vi "Search Results Panel.vi"(11 "BetterSearch in":refnum<class "BetterSearch.lvclass">) -> ()   [LabVIEW 2020, in "Better Search.lvlib" / "BetterSearch.lvclass"]
uses:
  BetterSearch.lvclass
  Search/Search.lvclass
  Data Types/Scope Options.ctl
  Data Types/Throbber.ctl
  BetterSearch.lvclass/BetterSearch.ctl
  80aabc45-af7a-4409-a262-2509359cf74b.vi
  Search Result/Search Result.lvclass
  Better Search.lvlib
panel:
  out "Throbber":T1
  out "Scope Options":T2
  in  "Results Table":i32[](listbox)
  out "Text":string
  out "Type":string
  in  "Go To":bool
  in  "Remove":bool
  out "Scope":string
  out "Launched From":string
  out "Current Search":refnum<class "Search.lvclass">
  # "Exclude"
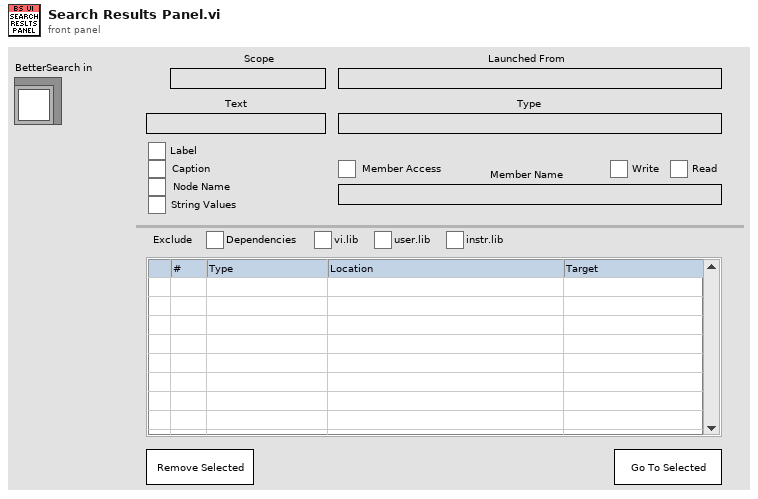
[diagram p1: front panel]
types:
  T1 = typedef "Better Search.lvlib/Throbber.ctl" = u16
  T2 = typedef "Better Search.lvlib/Scope Options.ctl" = cluster{"Include Labels":bool, "Include Captions":bool, "Include Node Name":bool, "Member Access":bool, "Member Read":bool, "Member Write":bool, "Member Name":string, "String Value":bool, "Dependencies":bool, "vi.lib":bool, "user.lib":bool, "instr.lib":bool}
  T3 = typedef "Better Search.lvlib/BetterSearch.lvclass/Results Events.ctl" = cluster{"Close Results Panel":refnum<user-event>, "Show Search":refnum<user-event>, "Show Result":refnum<user-event>, "Progress WD":refnum<user-event>}
  T4 = typedef "Better Search.lvlib/Search Params.ctl" = cluster{"Type":T5, "Type ID":string, "Text":string, "Scope":T6, "Targets":refnum<vi>[], "Scope Options":T2, "Typedef Path":path, "Member Graph Index":i32, "Member TypeID":string}
  T5 = typedef "Better Search.lvlib/Search Type.ctl" = enum16{"Generic", "Text", "Data Type", "VI", "Node"}
  T6 = typedef "Better Search.lvlib/Search Scope.ctl" = enum16{"Active Target", "Active Project", "Specific Targets", "Active VI", "Active Hierarchy"}
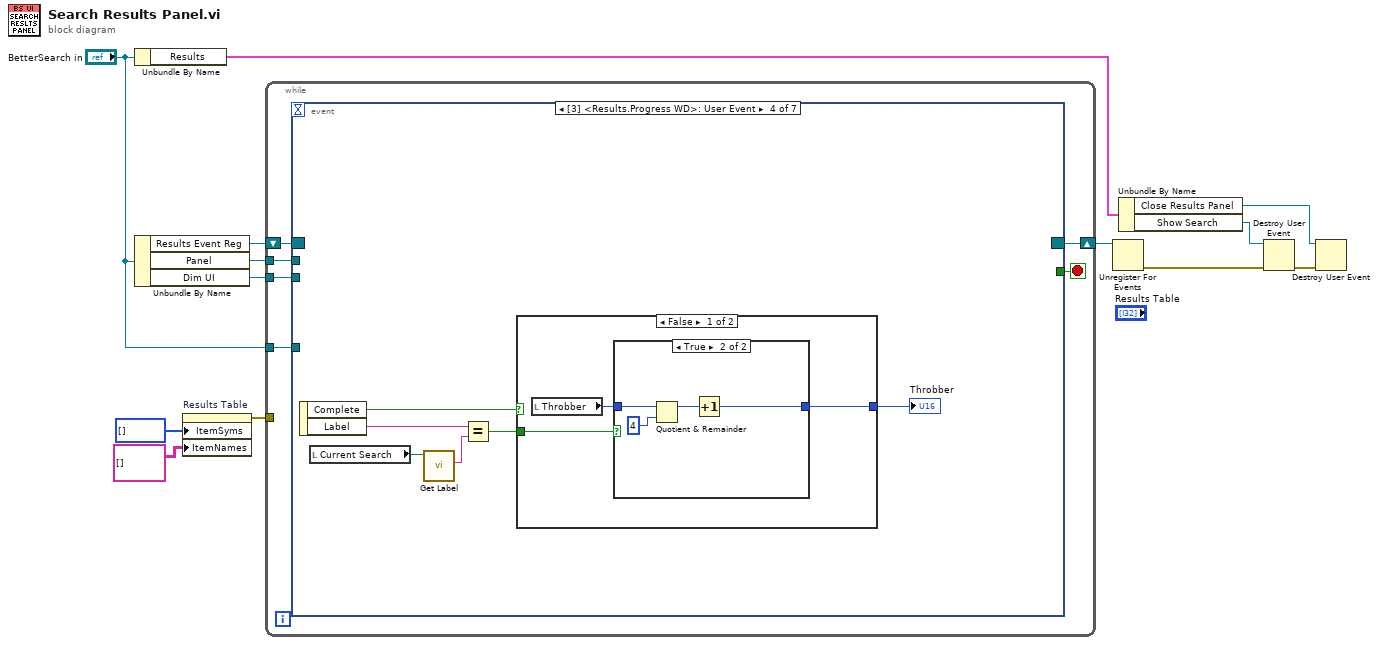
[diagram p0: block diagram]
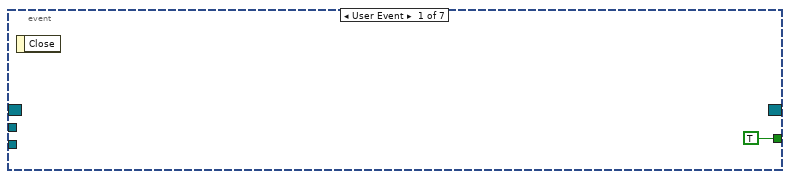
[diagram p2: hidden frame]
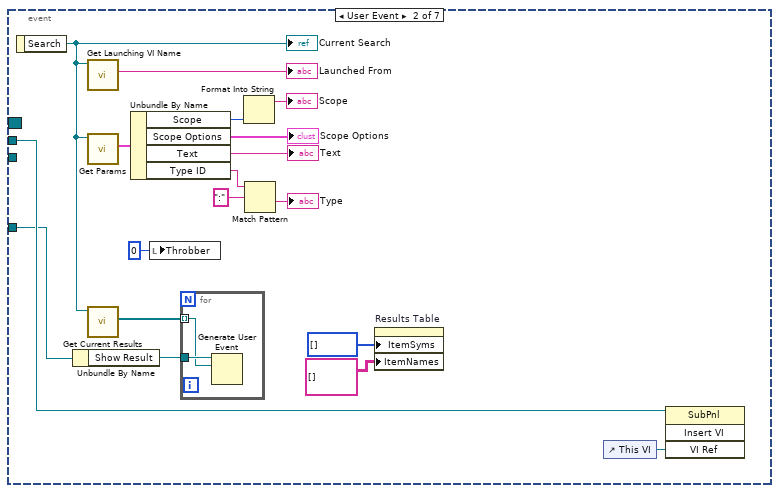
[diagram p3: hidden frame]
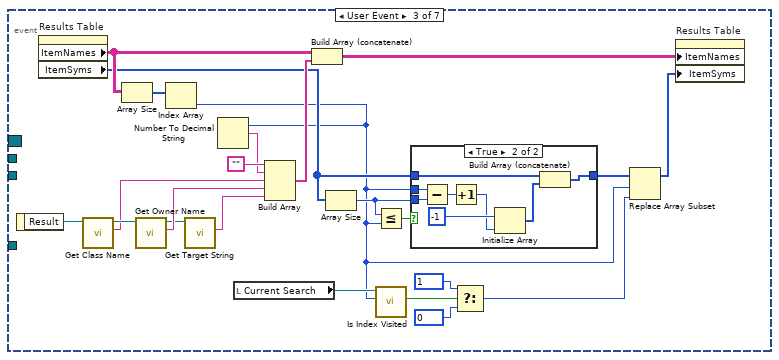
[diagram p4: hidden frame]
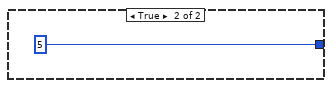
[diagram p7: hidden frame]
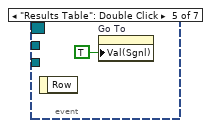
[diagram p8: hidden frame]
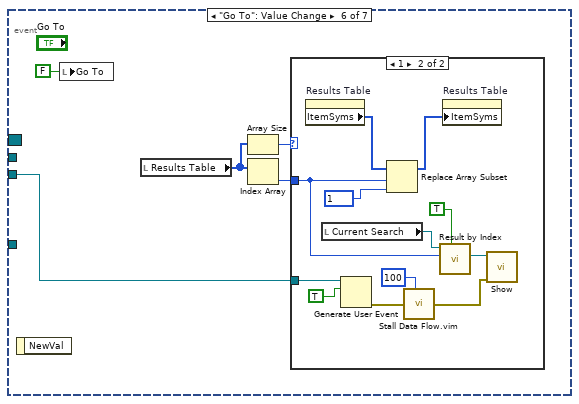
[diagram p9: hidden frame]
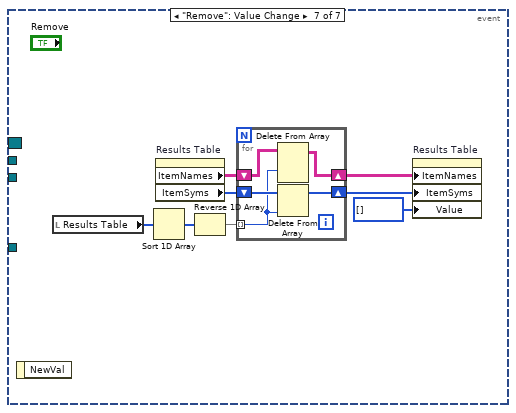
[diagram p11: hidden frame]
diagram:
  n1 = Unbundle By Name("BetterSearch in") -> ("Results"=w9:T3)
  n2 = Unbundle By Name("BetterSearch in") -> ("Results Event Reg"=w13:refnum<event-registration>, "Panel"=w6:refnum<vi>, "Dim UI"=w3:refnum<user-event>)
  n3 = property on="Results Table" class="MCListbox (strict)"("ItemSyms"=i32[] [] ("Item Symbols"), "ItemNames"=string[][] [] ("Item Names")) -> (error out=w2:errorcluster)  [unwired: 2 in, 1 out]
  n4 = while {
    shift-right: [w18] -> w12
    shift-left: w13 -> [w19]
    tunnel: w6 -> [w16]
    tunnel: w3 -> [w15]
    tunnel: w2 -> [_]
    tunnel: "BetterSearch in" -> [w14]
    stop <- w17 stop-if-true
    n5 = event shown="[3] <Results.Progress WD>: User Event" {
      selector: w19 -> [_ _ _ _ _ _ _]
      dyn-events: [_ _ _ _ _ _ _] -> w18
      timeout: _ -> [_ _ _ _ _ _ _]
      tunnel: [TRUE _ _ _ _ _ _] -> w17
      tunnel: w16 -> [_ w37 _ _ _ _ _]
      tunnel: w15 -> [_ _ _ _ _ w89 _]
      tunnel: w14 -> [_ w29 _ _ _ _ _]
      event User Event {
        n6 = event-data() -> ()  [unwired: 1 in, 1 out]
      }
      event User Event {
        n7 = event-data() -> ("Search"=w30:refnum<class "Search.lvclass">)  [unwired: 1 in]
        "Current Search" <- w30
        n8 = Unbundle By Name(w29) -> ("Show Result"=w28:refnum<user-event>)
        n9 = call "Get Launching VI Name.vi"("Search in"=w30) -> ("Launching VI Name"=→"Launched From":string)  [unwired: 8 in, 2 out]
        n10 = call "Get Params.vi"("Search in"=w30) -> ("Params"=w35:T4)  [unwired: 8 in, 2 out]
        n11 = call "Get Current Results.vi"("Search in"=w30) -> ("Current Results"=w27:refnum<class "Search Result.lvclass">[])  [unwired: 8 in, 2 out]
        n12 = Unbundle By Name(w35) -> ("Scope"=w34:T6, "Scope Options"=→"Scope Options":T2, "Text"=→"Text":string, "Type ID"=w25:string)
        n13 = local write "Throbber"(T1 0 ("Throbber")) -> ()
        n14 = for {
          tunnel: w28 -> [w40]
          tunnel: w27 -> [w39] mode=indexing
          n15 = Generate User Event(user event=w40, event data cluster=w39) -> ()  [unwired: 2 in, 2 out]
        }
        n16 = Format Into String(w34) -> (resulting string=→"Scope":string)  [unwired: 3 in, 1 out]
        n17 = Match Pattern(string=w25, regular expression=":") -> (after substring=→"Type":string)  [unwired: 1 in, 3 out]
        n18 = property on="Results Table" class="MCListbox (strict)"("ItemSyms"=i32[] [] ("Item Symbols"), "ItemNames"=string[][] [] ("Item Names")) -> ()  [unwired: 2 in, 2 out]
        n19 = control-ref of="This VI"() -> (w38:refnum<vi>)
        n20 = invoke class="SubPnl" method="Insert VI"(reference=w37, "VI Ref"=w38) -> ()  [unwired: 2 in, 4 out]
      }
      event User Event {
        n21 = event-data() -> ("Result"=w63:refnum<class "Search Result.lvclass">)  [unwired: 1 in]
        n22 = property on="Results Table" class="MCListbox (strict)"() -> ("ItemNames"=w56:string[][], "ItemSyms"=w49:i32[])  [unwired: 2 in, 2 out]
        n23 = call "Get Class Name.vi"("Search Result in"=w63) -> ("Class Name"=w61:string, "Search Result out"=w62:refnum<class "Search Result.lvclass">)  [unwired: 8 in, 1 out]
        n24 = Array Size(array=w56) -> (size(s)=w58:i32[])
        n25 = call "Get Owner Name.vi"("Search Result in"=w62) -> ("VI Name"=w60:string, "Search Result out"=w42:refnum<class "Search Result.lvclass">)  [unwired: 8 in, 1 out]
        n26 = Index Array(array=w58) -> (element=w43:i32)  [unwired: 1 in]
        n27 = call "Get Target String.vi"("Search Result in"=w42) -> ("Target"=w41:string)  [unwired: 8 in, 2 out]
        n28 = Number To Decimal String(number=w43) -> (decimal integer string=w57:string)  [unwired: 1 in]
        n29 = local read "Current Search"() -> (w53:refnum<class "Search.lvclass">)
        n30 = Build Array("", w57, w61, w60, w41) -> (w55:string[])
        n31 = Build Array (concatenate)(w56, w55) -> (w54:string[][])
        n32 = Array Size(array=w49) -> (size(s)=w48:i32)
        n33 = Less Or Equal?(x=w48, y=w43) -> (x <= y?=w50:bool)
        n34 = call "Is Index Visited.vi"("Index"=w43, "Search in"=w53) -> ("Visited?"=w52:bool)  [unwired: 7 in, 2 out]
        n35 = case shown="True" w50 {
          tunnel: w48 -> [_ w71]
          tunnel: w43 -> [_ w72]
          tunnel: w49 -> [w64 w69]
          tunnel: [w64 w67] -> w47
          frame False {
          }
          frame True {
            n36 = Subtract(x=w72, y=w71) -> (x-y=w70:i32)
            n37 = Increment(x=w70) -> (x+1=w65:i32)
            n38 = Initialize Array(-1, w65) -> (w68:i32[])
            n39 = Build Array (concatenate)(w69, w68) -> (w67:i32[])
          }
        }
        n40 = Select(t=1, s=w52, f=0) -> (s? t:f=w46:i32)
        n41 = Replace Array Subset(array=w47, new element=w46, index=w43) -> (w45:i32[])
        n42 = property on="Results Table" class="MCListbox (strict)"("ItemNames"=w54, "ItemSyms"=w45) -> ()  [unwired: 2 in, 2 out]
      }
      event User Event {
        n43 = event-data() -> ("Complete"=w75:bool, "Label"=w77:string)  [unwired: 1 in]
        n44 = local read "Current Search"() -> (w78:refnum<class "Search.lvclass">)
        n45 = call "Get Label.vi"("Search in"=w78) -> ("Label"=w76:string)  [unwired: 8 in, 2 out]
        n46 = Equal?(x=w77, y=w76) -> (x = y?=w74:bool)
        n47 = case shown="False" w75 {
          tunnel: w74 -> [w81 _]
          tunnel: [w79 T1 5 ("Throbber")] -> w73
          frame False {
            n48 = local read "Throbber"() -> (w80:T1)
            n49 = case shown="True" w81 {
              tunnel: w80 -> [w82 w86]
              tunnel: [w82 w83] -> w79
              frame False {
              }
              frame True {
                n50 = Quotient & Remainder(x=w86, y=T1 4) -> (x-y*floor(x/y)=w84:T1)  [unwired: 1 out]
                n51 = Increment(x=w84) -> (x+1=w83:T1)
              }
            }
          }
          frame True {
          }
        }
        "Throbber" <- w73
      }
      event "Results Table": Double Click {
        n52 = event-data() -> ()  [unwired: 1 in, 1 out]
        n53 = property on="Go To" class="Bool (strict)"("Val(Sgnl)"=TRUE ("Value (Signaling)")) -> ()  [unwired: 2 in, 2 out]
      }
      event "Go To": Value Change {
        n54 = event-data() -> ()  [unwired: 1 in, 1 out]
        n55 = local write "Go To"(FALSE ("Go To")) -> ()
        n56 = local read "Results Table"() -> (w92:i32[])
        n57 = Array Size(array=w92) -> (size(s)=w91:i32)
        n58 = Index Array(array=w92) -> (element=w90:i32)  [unwired: 1 in]
        n59 = case shown="1" w91 {
          tunnel: w90 -> [_ w101]
          tunnel: w89 -> [_ w99]
          frame 0, Default {
          }
          frame 1 {
            n60 = property on="Results Table" class="MCListbox (strict)"() -> ("ItemSyms"=w105:i32[])  [unwired: 2 in, 2 out]
            n61 = local read "Current Search"() -> (w102:refnum<class "Search.lvclass">)
            n62 = Generate User Event(user event=w99, event data cluster=TRUE ("event data")) -> (error out=w96:errorcluster)  [unwired: 2 in, 1 out]
            n63 = Replace Array Subset(array=w105, new element=1, index=w101) -> (w104:i32[])
            n64 = call "Stall Data Flow.vim"("value in"=w96, "milliseconds to wait"=u32 100) -> ("value out"=w95:errorcluster)  [unwired: 1 out]
            n65 = call "Result by Index.vi"("Mark Visited? (F)"=TRUE, "Result Index"=w101, "Search in"=w102) -> ("Result"=w100:refnum<class "Search Result.lvclass">)  [unwired: 6 in, 2 out]
            n66 = property on="Results Table" class="MCListbox (strict)"("ItemSyms"=w104) -> ()  [unwired: 2 in, 2 out]
            n67 = call "Show.vi"("error in (no error)"=w95, "Search Result in"=w100) -> ()  [unwired: 8 in, 2 out]
          }
        }
      }
      event "Remove": Value Change {
        n68 = event-data() -> ()  [unwired: 1 in, 1 out]
        n69 = local read "Results Table"() -> (w113:i32[])
        n70 = Sort 1D Array(array=w113) -> (sorted array=w112:i32[])
        n71 = property on="Results Table" class="MCListbox (strict)"() -> ("ItemNames"=w109:string[][], "ItemSyms"=w110:i32[])  [unwired: 2 in, 2 out]
        n72 = Reverse 1D Array(array=w112) -> (reversed array=w111:i32[])
        n73 = for {
          tunnel: w111 -> [w116] mode=indexing
          shift-right: [w114] -> w107
          shift-left: w110 -> [w118]
          shift-right: [w115] -> w108
          shift-left: w109 -> [w117]
          n74 = Delete From Array(array=w117, index (row)=w116) -> (array with subset deleted=w115:string[][])  [unwired: 2 in, 1 out]
          n75 = Delete From Array(array=w118, index=w116) -> (array with subset deleted=w114:i32[])  [unwired: 1 in, 1 out]
        }
        n76 = property on="Results Table" class="MCListbox (strict)"("ItemNames"=w108, "ItemSyms"=w107, "Value"=i32[] [] ("Results Table")) -> ()  [unwired: 2 in, 2 out]
      }
    }
  }
  n77 = Unregister For Events(event registration refnum=w12) -> (error out=w10:errorcluster)  [unwired: 1 in]
  n78 = Unbundle By Name(w9) -> ("Close Results Panel"=w7:refnum<user-event>, "Show Search"=w8:refnum<user-event>)
  n79 = Destroy User Event(user event=w8, error in=w10) -> (error out=w11:errorcluster)
  n80 = Destroy User Event(user event=w7, error in=w11) -> ()  [unwired: 1 out]
